vi "Download And Show Image From Website LV2012 NIVerfied.vi"() -> ()   [LabVIEW 2019]
doc: "This VI demonstrates how to download an image from a website and show it on the Frontpanel."
uses:
  <vilib>/httpClient/LabVIEWHTTPClient.lvlib
panel:
  out "Downloaded Image":picture
  in  "Image URL":string="http://forums.ni.com/legacyfs/online/20297_Labview-logo1.jpg"
  # "Overview: Demonstrates how to download an image from a website and show it on the Frontpanel. \nRequirements: LabVIEW Base Development System 2012 (or compatible)\nInstructions: \n1. Enter the URL of the image which you want to show.\n2. Run the VI."
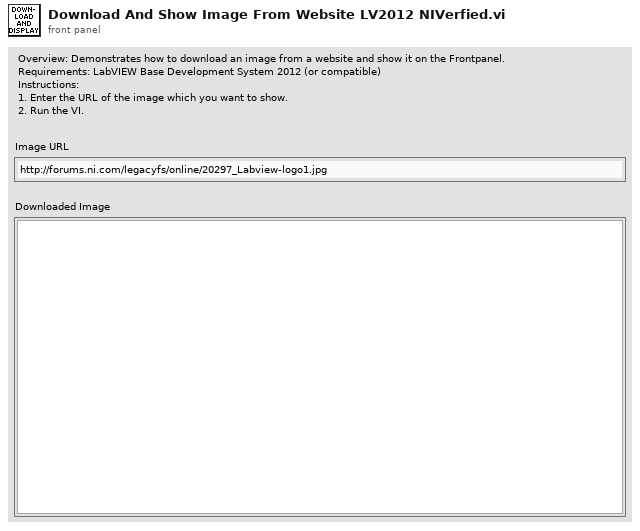
[diagram p1: front panel]
types:
  T1 = typedef "LabVIEWHTTPClient.lvlib/ClientHandle.ctl" = refnum<k1>
  T2 = typedef "imagedata.ctl" = cluster{"image type":i32, "image depth":i32, "image":u8[], "mask":u8[], "colors":u32[], "Rectangle":cluster{"left":i16, "top":i16, "right":i16, "bottom":i16}}
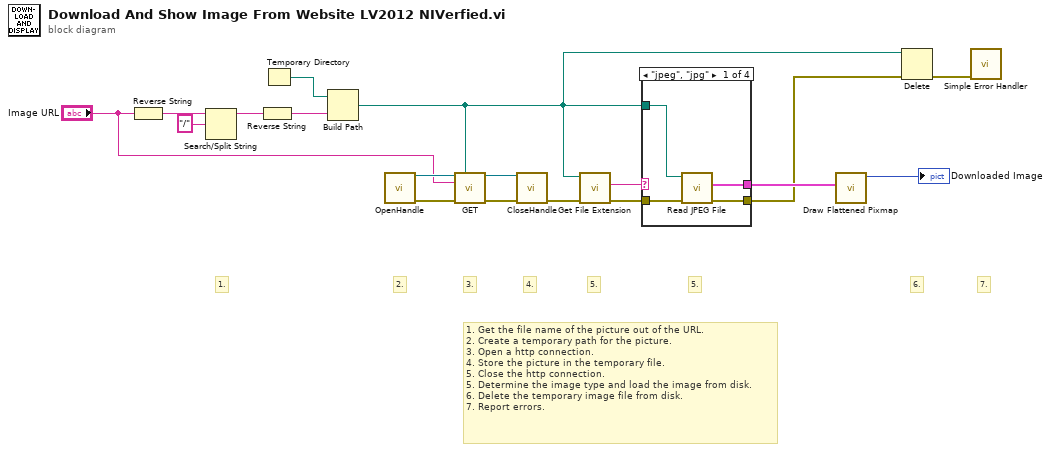
[diagram p0: block diagram]
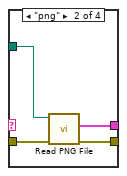
[diagram p2: hidden frame]
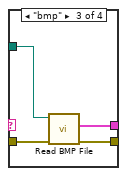
[diagram p3: hidden frame]
diagram:
  # "5."
  # "7."
  # "6."
  # "1. Get the file name of the picture out of the URL.\n2. Create a temporary path for the picture.\n3. Open a http connection.\n4. Store the picture in the temporary file.\n5. Close the http connection.\n5. Determine the image type and load the image from disk.\n6. Delete the temporary image file from disk.\n7. Report errors."
  # "5."
  # "4."
  # "3."
  # "2."
  # "1."
  n1 = Reverse String(1:"Image URL") -> (0:w9:string)
  n2 = Search/Split String(string=w9, search string/char (-)="/") -> (substring before match=w7:string)  [unwired: 1 in, 2 out]
  n3 = Reverse String(1:w7) -> (0:w6:string)
  n4 = Temporary Directory() -> (w12:path)
  n5 = Build Path(base path=w12, name or relative path=w6) -> (appended path=w3:path)
  n6 = call <vilib>:"OpenHandle.vi"() -> ("client handle out"=w18:T1, "error out"=w17:errorcluster)  [unwired: 14 in]
  n7 = call <vilib>:"GET.vi"("client handle"=w18, "output file"=w3, "url"="Image URL", "error in (no error)"=w17) -> ("client handle out"=w15:T1, "error out"=w16:errorcluster)  [unwired: 8 in, 2 out]
  n8 = call <vilib>:"CloseHandle.vi"("client handle"=w15, "error in (no error)"=w16) -> ("error out"=w11:errorcluster)  [unwired: 13 in]
  n9 = call <vilib>:"Get File Extension.vi"("error in (no error)"=w11, "file"=w3) -> ("error out"=w10:errorcluster, "lowercase file extension"=w13:string)  [unwired: 5 in, 3 out]
  n10 = case shown="\"jpeg\", \"jpg\"" w13 {
    tunnel: w3 -> [w21 w26 w27 _]
    tunnel: w10 -> [w22 w25 w30 w31]
    tunnel: [w20 w24 w29 w31] -> w5
    tunnel: [w19 w23 w28 _] -> w14
    frame "jpeg", "jpg" {
      n11 = call <vilib>:"Read JPEG File.vi"("error in (no error)"=w22, "path to JPEG file"=w21) -> ("error out"=w20:errorcluster, "image data"=w19:T2)  [unwired: 7 in, 1 out]
    }
    frame "png" {
      n12 = call <vilib>:"Read PNG File.vi"("error in (no error)"=w25, "path to PNG file"=w26) -> ("error out"=w24:errorcluster, "image data"=w23:T2)  [unwired: 7 in, 1 out]
    }
    frame "bmp" {
      n13 = call <vilib>:"Read BMP File.vi"("error in (no error)"=w30, "path to BMP file"=w27) -> ("error out"=w29:errorcluster, "image data"=w28:T2)  [unwired: 7 in, 1 out]
    }
    frame Default {
    }
  }
  n14 = call <vilib>:"Draw Flattened Pixmap.vi"("image data"=w14) -> ("new picture"=→"Downloaded Image":picture)  [unwired: 1 in, 7 out]
  n15 = Delete(path (use dialog)=w3, error in=w5) -> (error out=w4:errorcluster)  [unwired: 3 in, 2 out]
  n16 = call <vilib>:"Simple Error Handler.vi"("error in (no error)"=w4) -> ()  [unwired: 4 in, 5 out]
